vi "swerve-drive-pose-est-test.vi"(8 "error in (no error)":errorcluster) -> (0 "error out":errorcluster, 3 "Test Passed":bool)   [LabVIEW 2019]
uses:
  <vilib>/Rock Robotics/WPI/ThirdParty/JAS_Junk/TrajLib/TypeDef/ROTATION2D.ctl
  <vilib>/Rock Robotics/WPI/ThirdParty/JAS_Junk/TrajLib/MatBuilder_Create.vi
  <vilib>/Rock Robotics/WPI/ThirdParty/JAS_Junk/TrajLib/MatrixHelper_CoerceSize.vi
  <vilib>/Rock Robotics/WPI/ThirdParty/JAS_Junk/TrajLib/Util_CalcDist.vi
  <vilib>/Analysis/1siggen.llb/Gaussian White Noise.vi
  <vilib>/Rock Robotics/WPI/ThirdParty/JAS_Junk/TrajLib/Trajectory_Library.lvlib
panel:
  out "BenchProcessing Timer Per Pass":dbl
  out "BenchTotalTime":dbl
  out "BenchTotalPasses":dbl
  out "MaxErrPassed":bool
  out "TotalPassed":bool
  out "EerrSumNormalized":dbl
  out "Error Sum":dbl
  out "Max Error":dbl
  out "Using Vision":bool
  in  "UseVIsion":bool=TRUE
  out "VIsionUpdates":i32
  out "TotalTImeSecs":dbl
  out "Position Graph":cluster{dbl[], dbl[]}[](graph)
  out "PoesEstCreateErr":errorcluster
  # "< 0.125"
  # "< 0.05"
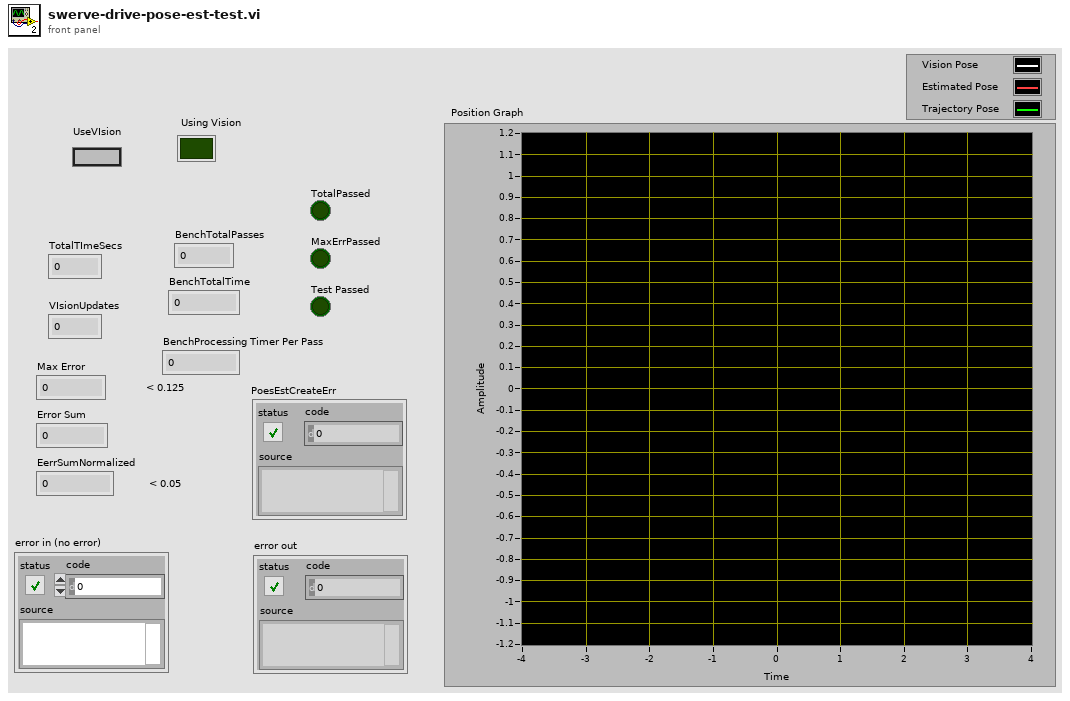
[diagram p1: front panel]
types:
  T1 = typedef "Trajectory_Library.lvlib/ROTATION2D.ctl" = cluster{"VALUE":dbl, "COS":dbl, "SIN":dbl}
  T2 = typedef "Trajectory_Library.lvlib/TRANSLATION2D.ctl" = cluster{"X":dbl, "Y":dbl}
  T3 = typedef "Trajectory_Library.lvlib/SWERVE_DRIVE_MODULE_POSITION.ctl" = cluster{"Distance":dbl, "Angle":T1, "P":bool}
  T4 = typedef "NI_Matrix.lvlib/RealMatrix.ctl" = dbl[][]
  T5 = typedef "Trajectory_Library.lvlib/POSE2D.ctl" = cluster{"TRANSLATION":T2, "ROTATION":T1}
  T6 = typedef "Trajectory_Library.lvlib/SWERVE_DRIVE_KINEMATICS.ctl" = cluster{"NumModules":i32, "InverseKinematics":T4, "ForwardKinematics":T4, "Modules":T2[], "PrevCoR":T2, "SavedModuleStates":T7[]}
  T7 = typedef "Trajectory_Library.lvlib/SWERVE_DRIVE_MODULE_STATE.ctl" = cluster{"Speed":dbl, "Angle":T1}
  T8 = typedef "Trajectory_Library.lvlib/TRAJ_CONFIG.ctl" = cluster{"MaxVelocity":dbl, "Max Acceleration":dbl, "StartVelocity":dbl, "End Velocity":dbl, "Reversed":bool, "Constraints":variant[]}
  T9 = typedef "Trajectory_Library.lvlib/SWERVE_DRIVE_POSE_EST.ctl" = cluster{"M_VisionContR":T4, "m_nominal_dT":dbl, "m_PrevTime_Sec":dbl, "m_GyroOffset":T1, "m_PrevAngle":T1, "m_Observer":T10, "m_kinematics":T6, "Pose_Buffer":T13, "States":i32, "Inputs":i32, "Outputs":i32}
  T10 = typedef "Trajectory_Library.lvlib/UNSCENTED_KALMAN_FILTER.ctl" = cluster{"m_P":T4, "m_xHat":T4, "States":i32, "Outputs":i32, "m_ContR":T4, "m_ContQ":T4, "m_SigmasF":T4, "m_dT_Sec":dbl, "MERWE_SCALED_SIGMA_PTS":T11, "meanFuncX":T12, "meanFuncY":T12, "residualFuncX":T12, "residualFuncY":T12, "addFuncX":T12, "addFuncXExtra":variant, "residualFuncYExtra":variant, "residualFuncXExtra":variant, "MeanFuncYExtra":variant, "MeanFuncXExtra":variant, "Inputs":i32}
  T11 = typedef "Trajectory_Library.lvlib/MERWE_SCALED_SIGMA_PTS.ctl" = cluster{"m_Wm":T4, "States":i32, "Alpha":dbl, "m_Wc":T4, "Kappa":i32}
  T12 = typedef "Trajectory_Library.lvlib/CALLBACK_FUNC_TYPE.ctl" = refnum<vi>
  T13 = typedef "Trajectory_Library.lvlib/TIME_INTERPOLATABLE_POSE2D.ctl" = cluster{"TimeStamps":dbl[], "Pose":T5[], "Min_TimeStamp":dbl, "Max_TimeStamp":dbl, "ItemCount":i32, "MaxBufferTime":dbl}
  T14 = typedef "Trajectory_Library.lvlib/TRAJECTORY.ctl" = cluster{"TotalTImeSecs":dbl, "States":T15[]}
  T15 = typedef "Trajectory_Library.lvlib/TRAJ_STATE.ctl" = cluster{"TimeSeconds":dbl, "Velocity":dbl, "Acceleration":dbl, "POSE":T5, "Curvature":dbl}
  T16 = typedef "Trajectory_Library.lvlib/CHASSIS_SPEEDS.ctl" = cluster{"vX":dbl, "vY":dbl, "vOmega":dbl}
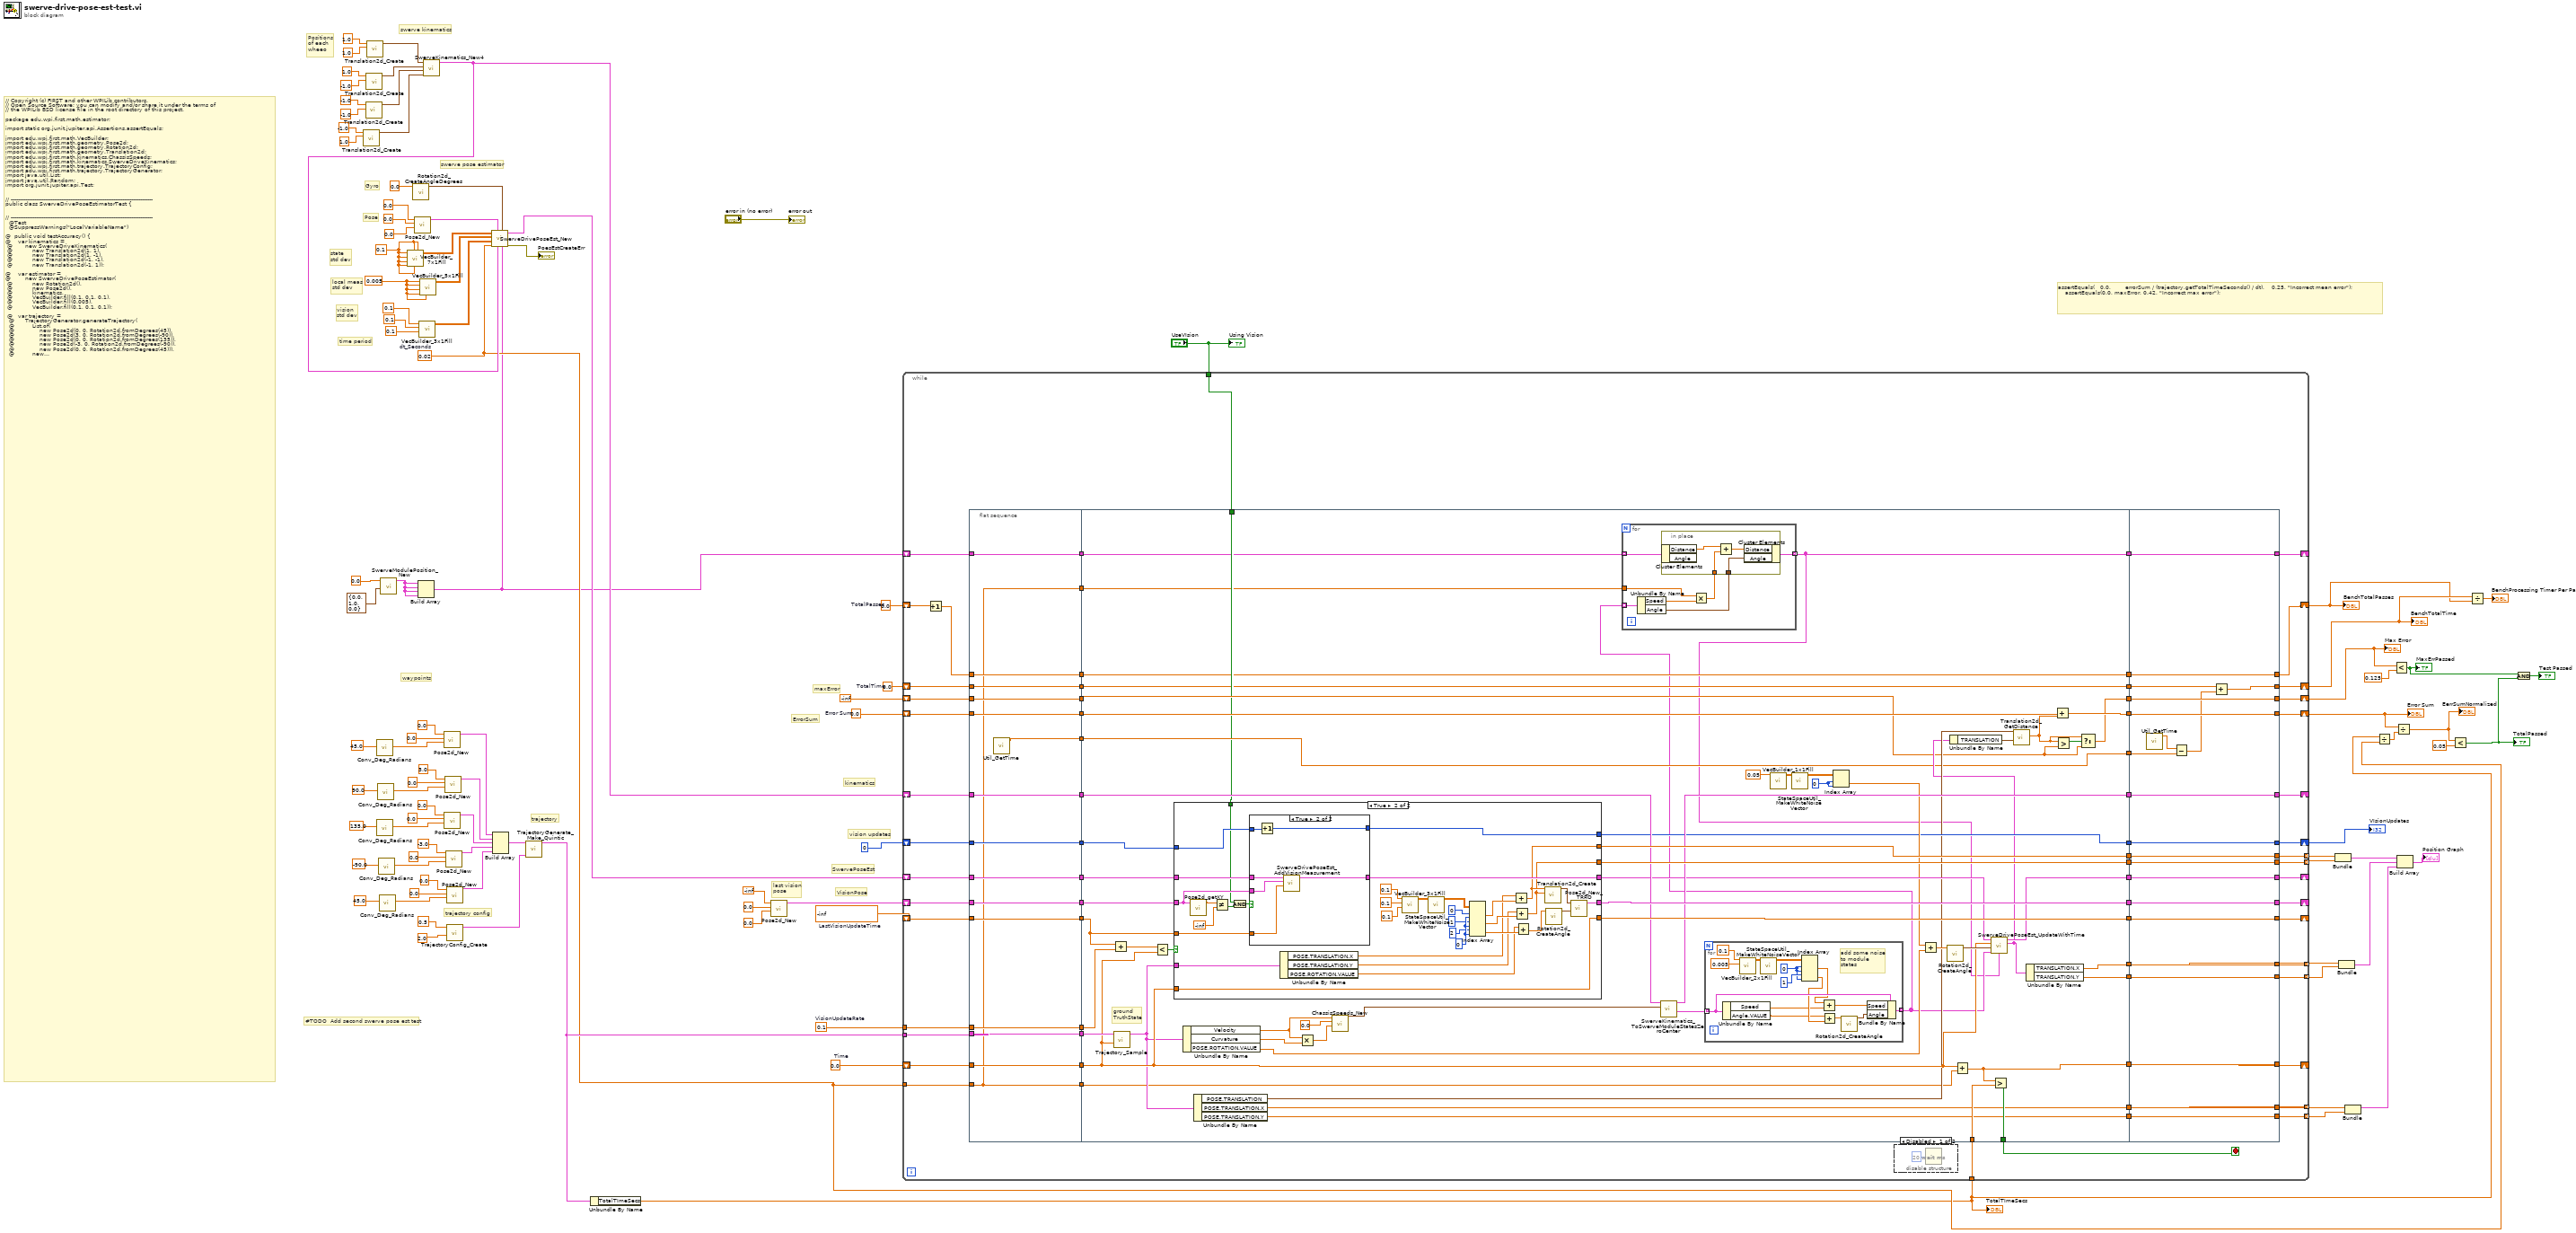
[diagram p0: block diagram]
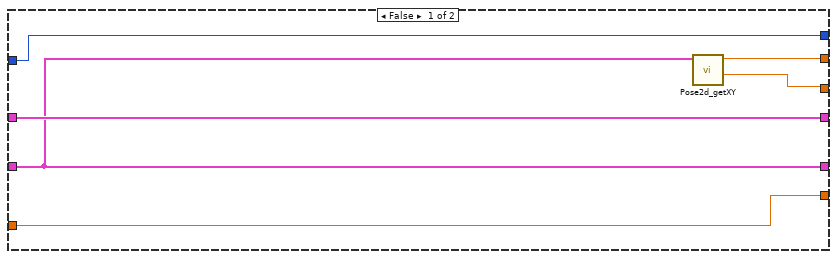
[diagram p3: hidden frame]
diagram:
  w12 = 0.0  # TotalPasses
  w13 = 0.0  # TotalTime
  w25 = 0.0  # Error Sum
  w45 = 0.1  # VisionUpdateRate
  w46 = -inf  # LastVisionUpdateTime
  w48 = 0.0  # Time
  w23 = 0.02  # dt_Seconds
  w2 = 0.005 ("element")
  w3 = 0.1 ("element")
  # "#TODO  Add second swerve pose est test"
  # "assertEquals(   0.0,        errorSum / (trajectory.getTotalTimeSeconds() / dt),    0.25, \"Incorrect mean error\");\n    assertEquals(0.0, maxError, 0.42, \"Incorrect max error\");"
  # "ErrorSum"
  # "maxError"
  # "vision updates"
  # "kinematics"
  # "SwervePoseEst"
  # "VisionPose"
  # "last vision\npose"
  # "time period"
  # "vision \nstd dev"
  # "local meas\nstd dev"
  # "state\nstd dev"
  # "Pose"
  # "Gyro"
  # "Positions\nof each\nwheeo"
  # "swerve pose estimator"
  # "swerve kinematics"
  # "trajectory config"
  # "trajectory"
  # "waypoints"
  # "// Copyright (c) FIRST and other WPILib contributors.\n// Open Source Software; you can modify and/or share it under the terms of\n// the WPILib BSD license file in the root directory of this project.\n\npackage edu.wpi.first.math.estimator;\n\nimport static org.junit.jupiter.api.Assertions.assertEquals;\n\nimport edu.wpi.first.math.VecBuilder;\nimport edu.wpi.first.math.geometry.Pose2d;\nimport edu.wpi.first.math.geometry.Rotation2d;\nimport edu.wpi.first.math.geometry.Translation2d;\nimport edu.wpi.first.math.kinematics.ChassisSpeeds;\nimport edu.wpi.first.math.kinematics.SwerveDriveKinematics;\nimport edu.wpi.first.math.trajectory.TrajectoryConfig;\nimport edu.wpi.first.math.trajectory.TrajectoryGenerator;\nimport java.util.List;\nimport java.util.Random;\nimport org.junit.jupiter.api.Test;\n\n\n// -------------------------------------------------------------------------------\npublic class SwerveDrivePoseEstimatorTest {\n\n\n// -------------------------------------------------------------------------------\n  @Test\n  @SuppressWarnings(\"LocalVariableName\")\n\n@  public void testAccuracy() {\n@    var kinematics =\n @       new SwerveDriveKinematics(\n @           new Translation2d(1, 1),\n @           new Translation2d(1, -1),\n @           new Translation2d(-1, -1),\n @           new Translation2d(-1, 1));\n\n@    var estimator =\n@        new SwerveDrivePoseEstimator(\n @           new Rotation2d(),\n @           new Pose2d(),\n @           kinematics,\n @           VecBuilder.fill(0.1, 0.1, 0.1),\n @           VecBuilder.fill(0.005),\n @           VecBuilder.fill(0.1, 0.1, 0.1));\n\n @   var trajectory =\n  @      TrajectoryGenerator.generateTrajectory(\n  @          List.of(\n  @              new Pose2d(0, 0, Rotation2d.fromDegrees(45)),\n  @              new Pose2d(3, 0, Rotation2d.fromDegrees(-90)),\n  @              new Pose2d(0, 0, Rotation2d.fromDegrees(135)),\n  @              new Pose2d(-3, 0, Rotation2d.fromDegrees(-90)),\n  @              new Pose2d(0, 0, Rotation2d.fromDegrees(45))),\n  @          new TrajectoryConfig(0.5, 2));\n\n    var rand = new Random(4915);\n\n@    final double dt = 0.02;\n @   double t = 0.0;\n\n @   final double visionUpdateRate = 0.1;\n  @  Pose2d lastVisionPose = null;\n @   double lastVisionUpdateTime = Double.NEGATIVE_INFINITY;\n\n @   double maxError = Double.NEGATIVE_INFINITY;\n  @  double errorSum = 0;\n\n@    while (t <= trajectory.getTotalTimeSeconds()) {\n\n @     var groundTruthState = trajectory.sample(t);\n\n @     if (lastVisionUpdateTime + visionUpdateRate < t) {\n  @      if (lastVisionPose != null) {\n   @       estimator.addVisionMeasurement(lastVisionPose, lastVisionUpdateTime);\n   @     }\n\n @       lastVisionPose =\n @           new Pose2d(\n @               new Translation2d(\n  @                  groundTruthState.poseMeters.getTranslation().getX() + rand.nextGaussian() * 0.1,\n  @                  groundTruthState.poseMeters.getTranslation().getY()\n  @                      + rand.nextGaussian() * 0.1),\n @               new Rotation2d(rand.nextGaussian() * 0.1)\n  @                  .plus(groundTruthState.poseMeters.getRotation()));\n\n  @      lastVisionUpdateTime = t;\n  @    }  // end if \n\n  @    var moduleStates =\n   @       kinematics.toSwerveModuleStates(\n    @          new ChassisSpeeds(\n     @             groundTruthState.velocityMetersPerSecond,\n      @            0.0,\n     @             groundTruthState.velocityMetersPerSecond\n    @                  * groundTruthState.curvatureRadPerMeter));\n\n @     for (var moduleState : moduleStates) {\n  @      moduleState.angle = moduleState.angle.plus(new Rotation2d(rand.nextGaussian() * 0.005));\n @       moduleState.speedMetersPerSecond += rand.nextGaussian() * 0.1;\n @     }\n\n\n @     var xHat =\n  @        estimator.updateWithTime(\n  @            t,\n  @            groundTruthState.poseMeters.getRotation()\n  @                .plus(new Rotation2d(rand.nextGaussian() * 0.05)),\n  @            moduleStates);\n\n @     double error =\n @         groundTruthState.poseMeters.getTranslation().getDistance(xHat.getTranslation());\n @     if (error > maxError) {\n  @      maxError = error;\n  @    }\n  @    errorSum += error;\n\n@      t += dt;\n @   }    // END OF LOOP\n\n    assertEquals(\n        0.0, errorSum / (trajectory.getTotalTimeSeconds() / dt), 0.25, \"Incorrect mean error\");\n    assertEquals(0.0, maxError, 0.42, \"Incorrect max error\");\n  }\n}"
  n1 = call <vilib>:"Translation2d_Create.vi"("Y"=1.0, "X"=-1.0) -> ("TRANSLATION"=w62:T2)  [unwired: 9 in]
  n2 = call <vilib>:"Translation2d_Create.vi"("Y"=-1.0, "X"=-1.0) -> ("TRANSLATION"=w63:T2)  [unwired: 9 in]
  n3 = call <vilib>:"Translation2d_Create.vi"("Y"=-1.0, "X"=1.0) -> ("TRANSLATION"=w64:T2)  [unwired: 9 in]
  n4 = call <vilib>:"Translation2d_Create.vi"("Y"=1.0, "X"=1.0) -> ("TRANSLATION"=w65:T2)  [unwired: 9 in]
  n5 = call <vilib>:"Conv_Deg_Radians.vi"("Degress"=45.0 ("Heading")) -> ("Radians"=w79:dbl)  [unwired: 10 in]
  n6 = call <vilib>:"Conv_Deg_Radians.vi"("Degress"=135.0 ("Heading")) -> ("Radians"=w87:dbl)  [unwired: 10 in]
  n7 = call <vilib>:"Conv_Deg_Radians.vi"("Degress"=90.0 ("Heading")) -> ("Radians"=w83:dbl)  [unwired: 10 in]
  n8 = call <vilib>:"Conv_Deg_Radians.vi"("Degress"=-90.0 ("Heading")) -> ("Radians"=w91:dbl)  [unwired: 10 in]
  n9 = call <vilib>:"Conv_Deg_Radians.vi"("Degress"=45.0 ("Heading")) -> ("Radians"=w95:dbl)  [unwired: 10 in]
  n10 = call <vilib>:"SwerveModulePosition_New.vi"("ROTATION"=T1 {"VALUE"=0.0, "COS"=1.0, "SIN"=0.0}, "Distance"=0.0) -> ("SWERVE_DRIVE_MODULE_POSITION"=w4:T3)  [unwired: 9 in]
  n11 = call <vilib>:"VecBuilder_7x1Fill.vi"("R0"=w3, "R6"=w3, "R1"=w3, "R5"=w3, "R4"=w3, "R3"=w3, "R2"=w3) -> ("output matrix"=w55:T4)  [unwired: 4 in]
  n12 = call <vilib>:"Rotation2d_CreateAngleDegrees.vi"("Angle_Degrees"=0.0) -> ("ROTATION"=w61:T1)  [unwired: 10 in]
  n13 = call <vilib>:"Pose2d_New.vi"("Heading"=0.0, "Y"=0.0, "X"=0.0) -> ("out POSe"=w59:T5)  [unwired: 8 in]
  n14 = Build Array(w4, w4, w4, w4) -> (w1:T3[])
  n15 = call <vilib>:"VecBuilder_3x1Fill.vi"("R2"=0.1 ("element"), "R1"=0.1 ("element"), "R0"=0.1 ("element")) -> ("output matrix"=w50:T4)  [unwired: 8 in]
  n16 = call <vilib>:"VecBuilder_5x1Fill.vi"("R4"=w2, "R3"=w2, "R2"=w2, "R1"=w2, "R0"=w2) -> ("output matrix"=w54:T4)  [unwired: 6 in]
  n17 = call <vilib>:"SwerveKinematics_New4.vi"("wheel 3"=w62, "wheel 2"=w63, "wheel 1"=w64, "wheel 0"=w65) -> ("SWERVE_DRIVE_KINEMATICS"=w38:T6)  [unwired: 7 in]
  n18 = call <vilib>:"Pose2d_New.vi"("Heading"=w79, "Y"=0.0, "X"=0.0) -> ("out POSe"=w78:T5)  [unwired: 8 in]
  n19 = call <vilib>:"Pose2d_New.vi"("Heading"=w87, "Y"=0.0, "X"=0.0) -> ("out POSe"=w75:T5)  [unwired: 8 in]
  n20 = call <vilib>:"Pose2d_New.vi"("Heading"=w83, "Y"=0.0, "X"=3.0) -> ("out POSe"=w76:T5)  [unwired: 8 in]
  n21 = call <vilib>:"Pose2d_New.vi"("Heading"=w91, "Y"=0.0, "X"=-3.0) -> ("out POSe"=w74:T5)  [unwired: 8 in]
  n22 = call <vilib>:"Pose2d_New.vi"("Heading"=w95, "Y"=0.0, "X"=0.0) -> ("out POSe"=w100:T5)  [unwired: 8 in]
  n23 = call <vilib>:"TrajectoryConfig_Create.vi"("MaxAcceleration"=2.0, "MaxVelocity"=0.5) -> ("TRAJECTORY_CONFIG"=w97:T8)  [unwired: 9 in]
  n24 = call <vilib>:"SwerveDrivePoseEst_New.vi"("ModulePositions"=w1, "gyroAngle"=w61, "SwerveKinematics"=w38, "InitialPose"=w59, "dt_Seconds"=w23, "VisionMeasurementStdDevs"=w50, "LocalMeasurementStdDevs"=w54, "StateStdDevs"=w55) -> ("Error"=→"PoesEstCreateErr":errorcluster, "SwerveDrivePoseEstimate"=w40:T9)  [unwired: 2 in]
  n25 = Build Array(w78, w76, w75, w74, w100) -> (w98:T5[])
  n26 = call <vilib>:"TrajectoryGenerate_Make_Quintic.vi"("traj_config"=w97, "waypointPOSE"=w98) -> ("TRAJECTORY"=w47:T14)  [unwired: 8 in, 1 out]
  n27 = Unbundle By Name(w47) -> ("TotalTImeSecs"=w16:dbl)
  "TotalTImeSecs" <- w16
  n28 = call <vilib>:"Pose2d_New.vi"("Heading"=0.0, "Y"=0.0, "X"=-inf) -> ("out POSe"=w41:T5)  [unwired: 8 in]
  n29 = while {
    tunnel: w23 -> [w115]
    shift-right: [w171] -> _
    shift-left: w48 -> [w158]
    tunnel: w47 -> [w169]
    tunnel: w16 -> [w170]
    shift-right: [w163] -> _
    shift-left: w46 -> [w165]
    tunnel: w45 -> [w168]
    shift-right: [w164] -> _
    shift-left: w41 -> [w167]
    shift-right: [w157] -> _
    shift-left: w40 -> [w166]
    tunnel: [w162] -> w39 mode=indexing
    tunnel: [w161] -> w37 mode=indexing
    shift-right: [w159] -> _
    shift-left: w38 -> [w160]
    tunnel: [w156] -> w36 mode=indexing
    tunnel: [w155] -> w35 mode=indexing
    shift-right: [w153] -> w30
    shift-left: 0 -> [w154]
    tunnel: [w152] -> w29 mode=indexing
    tunnel: [w151] -> w28 mode=indexing
    shift-right: [w148] -> w21
    shift-left: -inf -> [w147]
    shift-right: [w149] -> w24
    shift-left: w25 -> [w150]
    shift-right: [w118] -> w11
    shift-left: w13 -> [w112]
    shift-right: [w108] -> w10
    shift-left: w12 -> [w117]
    tunnel: "UseVIsion" -> [w116]
    shift-right: [w105] -> _
    shift-left: w1 -> [w106]
    stop <- w146 stop-if-true
    n30 = Increment(x=w117) -> (x+1=w109:dbl)
    n31 = flat-sequence {
      tunnel: w147 -> [w178]
      tunnel: w150 -> [w179]
      tunnel: w154 -> [w180]
      tunnel: w158 -> [w181]
      tunnel: w160 -> [w182]
      tunnel: w165 -> [w183]
      tunnel: w166 -> [w184]
      tunnel: w167 -> [w185]
      tunnel: w168 -> [w186]
      tunnel: w169 -> [w187]
      tunnel: w115 -> [w173]
      tunnel: [w173] -> w145
      tunnel: [w187] -> w144
      tunnel: [w186] -> w143
      tunnel: [w185] -> w142
      tunnel: [w184] -> w141
      tunnel: [w183] -> w140
      tunnel: [w182] -> w139
      tunnel: [w181] -> w138
      tunnel: [w180] -> w137
      tunnel: [w179] -> w136
      tunnel: [w178] -> w135
      tunnel: [w177] -> w120
      tunnel: [w176] -> w113
      tunnel: w112 -> [w176]
      tunnel: [w175] -> w110
      tunnel: w109 -> [w175]
      tunnel: [w174] -> w107
      tunnel: w106 -> [w174]
      tunnel: [w173] -> w103
      tunnel: [w245] -> w146
      tunnel: w170 -> [w243]
      tunnel: w145 -> [w192]
      tunnel: w144 -> [w242]
      tunnel: w143 -> [w240]
      tunnel: w142 -> [w238]
      tunnel: w141 -> [w237]
      tunnel: w140 -> [w236]
      tunnel: w139 -> [w226]
      tunnel: w138 -> [w214]
      tunnel: w137 -> [w210]
      tunnel: w136 -> [w202]
      tunnel: w135 -> [w197]
      tunnel: [w244] -> w134
      tunnel: [w235] -> w133
      tunnel: [w234] -> w132
      tunnel: [w233] -> w131
      tunnel: [w232] -> w130
      tunnel: [w225] -> w129
      tunnel: [w213] -> w128
      tunnel: [w212] -> w127
      tunnel: [w211] -> w126
      tunnel: [w209] -> w125
      tunnel: [w207] -> w124
      tunnel: [w206] -> w123
      tunnel: [w201] -> w122
      tunnel: [w198] -> w121
      tunnel: w120 -> [w196]
      tunnel: [w196] -> w119
      tunnel: w116 -> [w195]
      tunnel: [w194] -> w114
      tunnel: w113 -> [w194]
      tunnel: [w193] -> w111
      tunnel: w110 -> [w193]
      tunnel: w107 -> [w191]
      tunnel: [w188] -> w104
      tunnel: w103 -> [w190]
      tunnel: [w327] -> w148
      tunnel: [w328] -> w149
      tunnel: [w329] -> w151
      tunnel: [w330] -> w152
      tunnel: [w331] -> w153
      tunnel: [w332] -> w155
      tunnel: [w333] -> w156
      tunnel: [w334] -> w157
      tunnel: [w335] -> w159
      tunnel: [w336] -> w161
      tunnel: [w337] -> w162
      tunnel: [w338] -> w163
      tunnel: [w339] -> w164
      tunnel: [w340] -> w171
      tunnel: w134 -> [w340]
      tunnel: w133 -> [w339]
      tunnel: w132 -> [w338]
      tunnel: w131 -> [w337]
      tunnel: w130 -> [w336]
      tunnel: w129 -> [w335]
      tunnel: w128 -> [w334]
      tunnel: w127 -> [w333]
      tunnel: w126 -> [w332]
      tunnel: w125 -> [w331]
      tunnel: w124 -> [w330]
      tunnel: w123 -> [w329]
      tunnel: w122 -> [w328]
      tunnel: w121 -> [w327]
      tunnel: w119 -> [w325]
      tunnel: [w324] -> w118
      tunnel: w114 -> [w322]
      tunnel: [w321] -> w108
      tunnel: w111 -> [w321]
      tunnel: [w320] -> w105
      tunnel: w104 -> [w320]
      frame #0 {
        n32 = call <vilib>:"Util_GetTime.vi"() -> ("FPGA_Time_Seconds"=w177:dbl)  [unwired: 10 in, 1 out]
      }
      frame #1 {
        w219 = 0 ("index (col)")
        # "ground\nTruthState"
        n33 = Add(x=w236, y=w240) -> (x+y=w239:dbl)
        n34 = call <vilib>:"Trajectory_Sample.vi"("Time"=w214, "InputTRAJECTORY"=w242) -> ("OutputTRAJ_STATE"=w208:T15)  [unwired: 9 in]
        n35 = Less?(x=w239, y=w214) -> (x < y?=w241:bool)
        n36 = case shown="True" w241 {
          tunnel: w238 -> [w275 w308]
          tunnel: w237 -> [w277 w309]
          tunnel: [w277 w307] -> w223
          tunnel: w236 -> [w276 w306]
          tunnel: w208 -> [_ w299]
          tunnel: [w275 w305] -> w235
          tunnel: w214 -> [_ w285]
          tunnel: [w276 w285] -> w234
          tunnel: [w274 w284] -> w233
          tunnel: [w273 w283] -> w232
          tunnel: w210 -> [w272 w282]
          tunnel: [w272 w281] -> w209
          tunnel: w195 -> [_ w278]
          frame False {
            n37 = call <vilib>:"Pose2d_getXY.vi"("in POSE"=w275) -> ("Y"=w273:dbl, "X"=w274:dbl)  [unwired: 9 in]
          }
          frame True {
            w296 = 0 ("index (col)")
            n38 = call <vilib>:"Pose2d_getXY.vi"("in POSE"=w308) -> ("X"=w311:dbl)  [unwired: 9 in, 1 out]
            n39 = Not Equal?(x=w311, y=-inf) -> (x != y?=w279:bool)
            n40 = And(x=w278, y=w279) -> (x .and. y?=w280:bool)
            n41 = case shown="True" w280 {
              tunnel: w309 -> [w313 w319]
              tunnel: w308 -> [_ w318]
              tunnel: [w313 w317] -> w307
              tunnel: w306 -> [_ w316]
              tunnel: w282 -> [w312 w315]
              tunnel: [w312 w314] -> w281
              frame False {
              }
              frame True {
                n42 = Increment(x=w315) -> (x+1=w314:i32)
                n43 = call <vilib>:"SwerveDrivePoseEst_AddVisionMeasurement.vi"("TImeStamp_Seconds"=w316, "visionRobotPose"=w318, "in SwerveDrivePoseEstimate"=w319) -> ("OutSwerveDrivePoseEstimate"=w317:T9)  [unwired: 7 in, 1 out]
              }
            }
            n44 = Unbundle By Name(w299) -> ("POSE.TRANSLATION.X"=w288:dbl, "POSE.TRANSLATION.Y"=w287:dbl, "POSE.ROTATION.VALUE"=w286:dbl)
            n45 = call <vilib>:"VecBuilder_3x1Fill.vi"("R2"=0.1, "R1"=0.1, "R0"=0.1) -> ("output matrix"=w303:T4)  [unwired: 8 in]
            n46 = call <vilib>:"StateSpaceUtil_MakeWhiteNoiseVector.vi"("StdDevs"=w303) -> ("WhiteNoise"=w297:T4)  [unwired: 9 in, 1 out]
            n47 = Index Array(array=w297, index (row) #1=0 ("index (col)"), index (col) #1=w296, index (row) #2=1 ("index (col)"), index (col) #2=w296, index (row) #3=2 ("index (col)"), index (col) #3=w296) -> (element #1=w290:dbl, element #2=w291:dbl, element #3=w292:dbl)
            n48 = Add(x=w288, y=w290) -> (x+y=w284:dbl)
            n49 = Add(x=w287, y=w291) -> (x+y=w283:dbl)
            n50 = Add(x=w286, y=w292) -> (x+y=w289:dbl)
            n51 = call <vilib>:"Translation2d_Create.vi"("Y"=w283, "X"=w284) -> ("TRANSLATION"=w304:T2)  [unwired: 9 in]
            n52 = call <vilib>:"Rotation2d_CreateAngle.vi"("Angle"=w289) -> ("ROTATION"=w298:T1)  [unwired: 10 in]
            n53 = call <vilib>:"Pose2d_New_TRRO.vi"("ROTATION"=w298, "TRANSLATION"=w304) -> ("outPOSE"=w305:T5)  [unwired: 9 in]
          }
        }
        n54 = Unbundle By Name(w208) -> ("Velocity"=w229:dbl, "Curvature"=w230:dbl, "POSE.ROTATION.VALUE"=w218:dbl)
        n55 = Unbundle By Name(w208) -> ("POSE.TRANSLATION"=w205:T2, "POSE.TRANSLATION.X"=w206:dbl, "POSE.TRANSLATION.Y"=w207:dbl)
        n56 = Multiply(x=w229, y=w230) -> (x*y=w228:dbl)
        n57 = call <vilib>:"ChassisSpeeds_New.vi"("vAngular"=w228, "vY"=0.0, "vX"=w229) -> ("CHASSIS"=w227:T16)  [unwired: 8 in]
        n58 = call <vilib>:"SwerveKinematics_ToSwerveModuleStatesZeroCenter.vi"("ChassisSpeeds"=w227, "in SWERVE_DRIVE_KINEMATICS"=w226) -> ("ModuleStates"=w224:T7[], "out SWERVE_DRIVE_KINEMATICS"=w225:T6)  [unwired: 8 in]
        n59 = for {
          tunnel: w224 -> [w265] mode=indexing
          tunnel: [w257] -> w189 mode=indexing
          w266 = 0 ("index (col)")
          # "add some noise\nto module\nstates"
          n60 = Unbundle By Name(w265) -> ("Speed"=w259:dbl, "Angle.VALUE"=w258:dbl)
          n61 = call <vilib>:"VecBuilder_2x1Fill.vi"("R1"=0.005, "R0"=0.1) -> ("output matrix"=w271:T4)  [unwired: 9 in]
          n62 = call <vilib>:"StateSpaceUtil_MakeWhiteNoiseVector.vi"("StdDevs"=w271) -> ("WhiteNoise"=w268:T4)  [unwired: 9 in, 1 out]
          n63 = Index Array(array=w268, index (row) #1=w266, index (col) #1=w266, index (row) #2=1 ("index (col)"), index (col) #2=w266) -> (element #1=w260:dbl, element #2=w261:dbl)
          n64 = Add(x=w260, y=w259) -> (x+y=w262:dbl)
          n65 = Add(x=w258, y=w261) -> (x+y=w263:dbl)
          n66 = call <vilib>:"Rotation2d_CreateAngle.vi"("Angle"=w263) -> ("ROTATION"=w264:T1)  [unwired: 10 in]
          n67 = Bundle By Name(cluster=w265, "Speed"=w262, "Angle"=w264) -> (w257:T7)
        }
        n68 = for {
          tunnel: w191 -> [w248] mode=indexing
          tunnel: w189 -> [w252] mode=indexing
          tunnel: [w247] -> w188 mode=indexing
          tunnel: w190 -> [w246]
          n69 = Unbundle By Name(w252) -> ("Speed"=w250:dbl, "Angle"=w251:T1)
          n70 = Multiply(x=w246, y=w250) -> (x*y=w249:dbl)
          n71 = in-place {
            in-place-border: w251 -> [w256]
            in-place-border: w249 -> [w254]
            n72 = in-place-cluster #1(w248) -> ("Distance"=w255:dbl)  [unwired: 1 out]
            n73 = Add(x=w255, y=w254) -> (x+y=w253:dbl)
            n74 = in-place-cluster #1("Distance"=w253, "Angle"=w256) -> (w247:T3)
          }
        }
        n75 = call <vilib>:"VecBuilder_1x1Fill.vi"("R0_C0"=0.05 ("R0")) -> ("output matrix"=w222:T4)  [unwired: 10 in]
        n76 = call <vilib>:"StateSpaceUtil_MakeWhiteNoiseVector.vi"("StdDevs"=w222) -> ("WhiteNoise"=w220:T4)  [unwired: 9 in, 1 out]
        n77 = Index Array(array=w220, index (row)=w219, index (col)=w219) -> (element=w217:dbl)
        n78 = Add(x=w217, y=w218) -> (x+y=w216:dbl)
        n79 = call <vilib>:"Rotation2d_CreateAngle.vi"("Angle"=w216) -> ("ROTATION"=w215:T1)  [unwired: 10 in]
        n80 = Add(x=w214, y=w192) -> (x+y=w244:dbl)
        n81 = call <vilib>:"SwerveDrivePoseEst_UpdateWithTime.vi"("ModulePositions"=w188, "SweveModuleStates"=w189, "GyroAngle"=w215, "CurrentTimeSeconds"=w214, "in SwerveDrivePoseEstimate"=w223) -> ("Estimated Pose"=w204:T5, "Out SwerveDrivePoseEstimate"=w213:T9)  [unwired: 4 in, 1 out]
        n82 = Unbundle By Name(w204) -> ("TRANSLATION"=w203:T2)
        n83 = Greater?(x=w244, y=w243) -> (0:w245:bool)
        n84 = call <vilib>:"Translation2d_GetDistance.vi"("other Translation"=w203, "In Translation"=w205) -> ("Distance"=w199:dbl)  [unwired: 9 in]
        n85 = Unbundle By Name(w204) -> ("TRANSLATION.X"=w212:dbl, "TRANSLATION.Y"=w211:dbl)
        n86 = Add(x=w202, y=w199) -> (x+y=w201:dbl)
        n87 = Greater?(x=w199, y=w197) -> (0:w200:bool)
        n88 = Select(t=w199, s=w200, f=w197) -> (s? t:f=w198:dbl)
      }
      frame #2 {
        n89 = call <vilib>:"Util_GetTime.vi"() -> ("FPGA_Time_Seconds"=w326:dbl)  [unwired: 10 in, 1 out]
        n90 = Subtract(x=w326, y=w325) -> (x-y=w323:dbl)
        n91 = Add(x=w322, y=w323) -> (x+y=w324:dbl)
      }
    }
    n92 = disable-structure shown="Disabled" {
      frame Disabled {
        n93 = Wait (ms)(milliseconds to wait=u32 20) -> ()  [unwired: 1 out]
      }
      frame Enabled {
      }
    }
  }
  "VIsionUpdates" <- w30
  "Max Error" <- w21
  "Error Sum" <- w24
  "BenchTotalPasses" <- w10
  "BenchTotalTime" <- w11
  n94 = Bundle(w39, w37) -> (w34:cluster{dbl[], dbl[]})  [unwired: 1 in]
  n95 = Bundle(w36, w35) -> (w33:cluster{dbl[], dbl[]})  [unwired: 1 in]
  n96 = Bundle(w28, w29) -> (w27:cluster{dbl[], dbl[]})  [unwired: 1 in]
  n97 = Divide(x=w16, y=w23) -> (x/y=w14:dbl)
  n98 = Less?(x=w21, y=0.125) -> (x < y?=w19:bool)
  "MaxErrPassed" <- w19
  n99 = Divide(x=w24, y=w14) -> (x/y=w15:dbl)
  "EerrSumNormalized" <- w15
  n100 = Build Array(w34, w33, w27) -> (→"Position Graph":cluster{dbl[], dbl[]}[])
  n101 = Less?(x=w15, y=0.05) -> (x < y?=w18:bool)
  "TotalPassed" <- w18
  n102 = Divide(x=w11, y=w10) -> (x/y=→"BenchProcessing Timer Per Pass":dbl)
  n103 = And(x=w19, y=w18) -> (x .and. y?=→"Test Passed":bool)
  "Using Vision" <- "UseVIsion"
  "error out" <- "error in (no error)"
